vi "test Send from Listener.vi"(8 "error in (no error)":errorcluster, 11 "TestCase in":refnum<class "Test Network Stream Nested Endpoint.lvclass">) -> (0 "error out":errorcluster, 3 "TestCase out":refnum<class "Test Network Stream Nested Endpoint.lvclass">)   [LabVIEW 2020, in "Test Network Stream Nested Endpoint.lvclass"]
uses:
  Test Network Stream Nested Endpoint.lvclass
  <vilib>/addons/_JKI Toolkits/VI Tester/TestCase.llb/TestCase.lvclass
  <vilib>/ActorFramework/Message Queue/Message Queue.lvclass
  <vilib>/ActorFramework/Message Dequeuer/Message Dequeuer.lvclass
  <vilib>/ActorFramework/Message Enqueuer/Message Priority.ctl
  <vilib>/ActorFramework/Message Enqueuer/Message Enqueuer.lvclass
  Support/String Data Msg/String Data Msg.lvclass
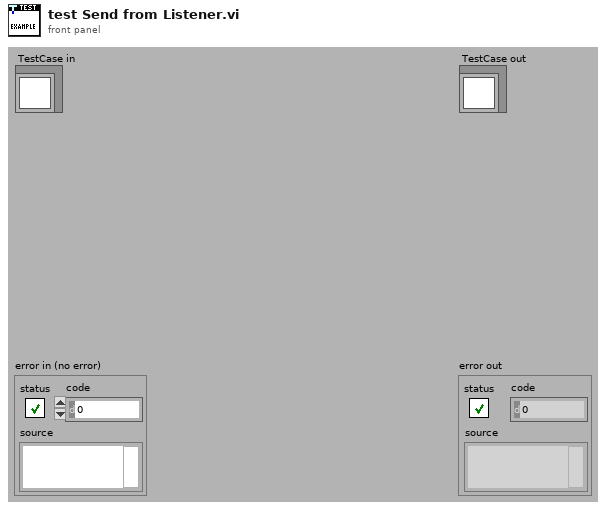
[diagram p1: front panel]
types:
  T1 = typedef "Actor Framework.lvlib/Message Enqueuer.lvclass/Message Priority.ctl" = enum16{"Low", "Normal", "High"}
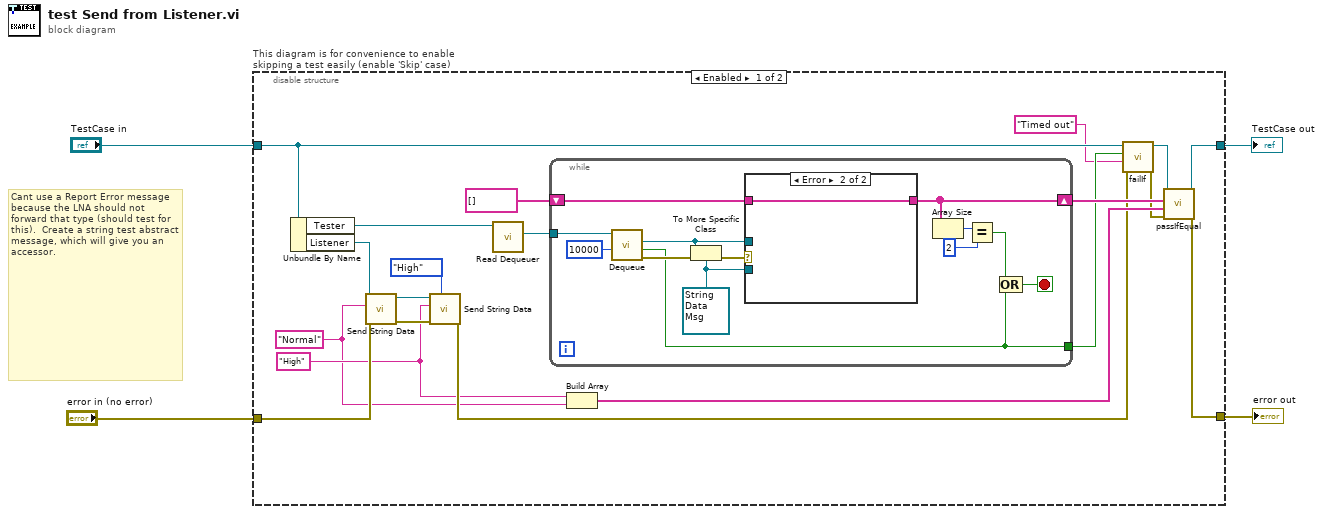
[diagram p0: block diagram]
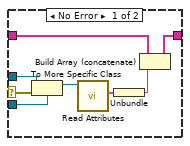
[diagram p2: hidden frame]
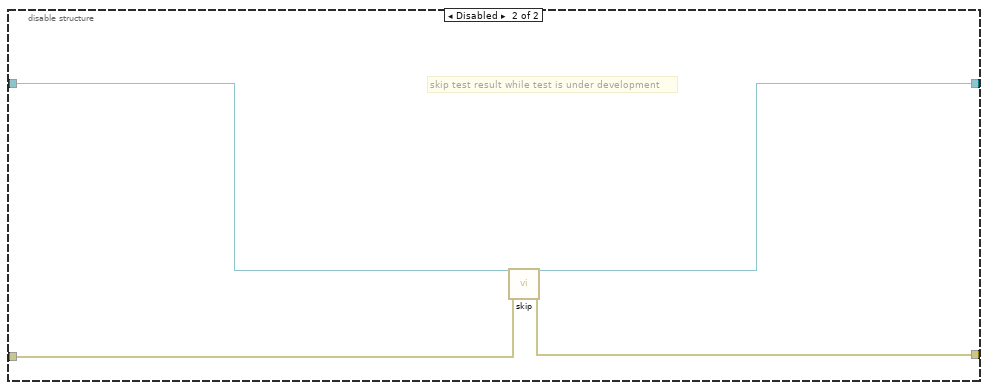
[diagram p3: hidden frame]
diagram:
  # "Cant use a Report Error message because the LNA should not forward that type (should test for this).  Create a string test abstract message, which will give you an accessor."
  n1 = disable-structure "This diagram is for convenience to enable skipping a test easily (enable 'Skip' case)" shown="Enabled" {
    disable-tunnel: "TestCase in" -> [w17 w50]
    disable-tunnel: [w24 w48] -> w1
    disable-tunnel: [w23 w49] -> w3
    disable-tunnel: "error in (no error)" -> [w9 w47]
    frame Enabled {
      w7 = "High" ("source")
      w6 = "Normal" ("source")
      n2 = Unbundle By Name(w17) -> ("Tester"=w21:refnum<class "Message Queue.lvclass">, "Listener"=w12:refnum<class "Message Enqueuer.lvclass">)
      n3 = call "Send String Data.vi"("error in (no error)"=w9, "String"=w6, "Message Enqueuer"=w12) -> ("error out"=w10:errorcluster, "Message Enqueuer out"=w11:refnum<class "Message Enqueuer.lvclass">)  [unwired: 7 in]
      n4 = call "Send String Data.vi"("Message Priority (Normal)"=Message_Priority."High", "error in (no error)"=w10, "String"=w7, "Message Enqueuer"=w11) -> ("error out"=w8:errorcluster)  [unwired: 6 in, 1 out]
      n5 = call <vilib>:"Read Dequeuer.vi"("Message Queue"=w21) -> ("Message Dequeuer"=w22:refnum<class "Message Dequeuer.lvclass">)  [unwired: 10 in]
      n6 = while {
        tunnel: w22 -> [w37]
        shift-right: [w30] -> w19
        shift-left: string[] [] -> [w31]
        tunnel: [w26] -> w15
        stop <- w34 stop-if-true
        w25 = refnum<class "String Data Msg.lvclass"> refnum ("String Data Msg.lvclass")
        n7 = call <vilib>:"Dequeue.vi"("timeout in ms (-1)"=10000, "Message Dequeuer in"=w37) -> ("error out"=w35:errorcluster, "timed out?"=w26:bool, "Message"=w32:refnum<class "Message.lvclass">)  [unwired: 5 in, 2 out]
        n8 = To More Specific Class(target class=w25, reference=w32, error in=w35) -> (error out=w33:errorcluster)  [unwired: 1 out]
        n9 = case shown="Error" w33 {
          selector: w33 -> [w45 _]
          tunnel: w32 -> [w44 _]
          tunnel: w25 -> [w43 _]
          tunnel: w31 -> [w42 w46]
          tunnel: [w41 w46] -> w30
          frame No Error {
            n10 = To More Specific Class(target class=w43, reference=w44, error in=w45) -> (specific class reference=w40:refnum<class "String Data Msg.lvclass">)  [unwired: 1 out]
            n11 = call "Read Attributes.vi"("Abstract Message Template in"=w40) -> ("Payload"=w39:cluster{"String":string})  [unwired: 9 in, 1 out]
            n12 = Unbundle(w39) -> ("String"=w38:string)
            n13 = Build Array (concatenate)(w42, w38) -> (w41:string[])
          }
          frame Error {
          }
        }
        n14 = Array Size(array=w30) -> (size(s)=w29:i32)
        n15 = Equal?(x=w29, y=2) -> (x = y?=w27:bool)
        n16 = Compound Arithmetic op=OR(w27, w26) -> (w34:bool)
      }
      n17 = Build Array(w7, w6) -> (w18:string[])
      n18 = call-dynamic "failIf.vi"("error in (no error)"=w8, "message (\"\")"="Timed out" ("message (\"\")"), "fail"=w15, "TestCase in"=w17) -> ("error out"=w14:errorcluster, "TestCase out"=w16:refnum<class "Test Network Stream Nested Endpoint.lvclass">)  [unwired: 6 in]
      n19 = call-dynamic "passIfEqual.vi"("error in (no error)"=w14, "y"=w18, "x"=w19, "TestCase in"=w16) -> ("error out"=w23:errorcluster, "TestCase out"=w24:refnum<class "Test Network Stream Nested Endpoint.lvclass">)  [unwired: 6 in]
    }
    frame Disabled {
      # "skip test result while test is under development"
      n20 = call <vilib>:"skip.vi"("error in (no error)"=w47, "TestCase in"=w50) -> ("error out"=w49:errorcluster, "TestCase out"=w48:refnum<class "Test Network Stream Nested Endpoint.lvclass">)  [unwired: 8 in]
    }
  }
  "error out" <- w3
  "TestCase out" <- w1
